vi "Immediate but left and right.vi"(7 "Description":string, 8 "Command Info In":T1, 9 "Right Speed":dbl, 10 "Left Speed":dbl) -> (0 "Command Info Out":T1)   [LabVIEW 2018]
doc: "This template is useful for immediate subsystem actions that do not need deadband filtering\n\nBe sure to right-click and select New from Template and save with a new command name."
uses:
  <vilib>/Rock Robotics/WPI/Framework/Command Status Info.ctl
  <vilib>/Rock Robotics/WPI/Framework/Completion Status.ctl
  <vilib>/Rock Robotics/WPI/Framework/Completion Notifier.ctl
  Implementation/Intake Operations.ctl
  Implementation/Intake Setpoints.ctl
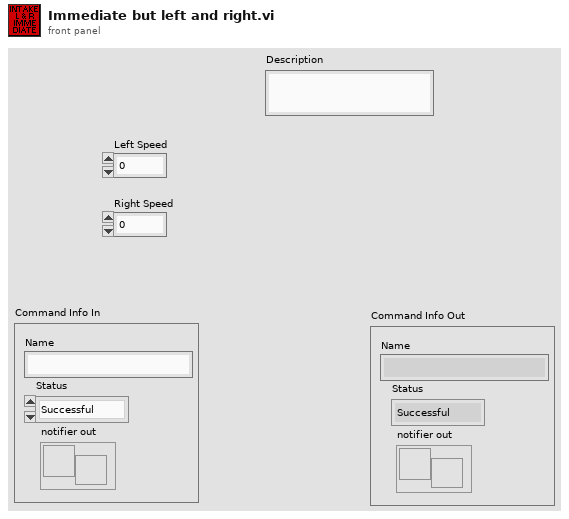
[diagram p1: front panel]
types:
  T1 = typedef "Command Status Info.ctl" = cluster{"Name":string, "Status":T2, "notifier out":T3}
  T2 = typedef "Completion Status.ctl" = enum16{"Successful", "Aborted", "Incomplete"}
  T3 = typedef "Completion Notifier.ctl" = refnum<notifier>
  T4 = typedef "Intake Operations.ctl" = enum16{"Reserve", "Read Current", "Immediate", "Intake for Duration", "Intake Until Cube"}
  T5 = typedef "Intake Setpoints.ctl" = cluster{"Operation":T4, "Left Speed":dbl, "Duration":dbl, "Right Speed":dbl}
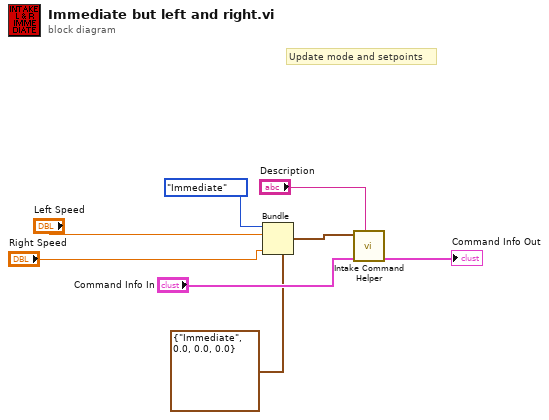
[diagram p0: block diagram]
diagram:
  # "Update mode and setpoints"
  n1 = Bundle(cluster=T5 {"Operation"=enum."Immediate", "Left Speed"=0.0, "Duration"=0.0, "Right Speed"=0.0} ("SubSystem Data"), "Operation"=Intake_Operations."Immediate", "Left Speed"="Left Speed", "Right Speed"="Right Speed") -> (w4:T5)  [unwired: 1 in]
  n2 = call "Intake Command Helper.vi"("Description"="Description", "Command Info In"="Command Info In", "SubSystem Data"=w4) -> ("Command Info Out"=→"Command Info Out":T1)  [unwired: 6 in, 2 out]
